vi "move calc rotation.vi"(8 "error in (no error)":errorcluster, 9 "New Value":dbl, 10 "Old Value":dbl) -> (0 "error out":errorcluster, 2 "Direction":bool=TRUE, 3 "steps":i32, 4 "Degrees":i32, 5 "rotate direction":string)   [LabVIEW 2014, in "AISAS motor.lvclass"]
uses:
  AISAS motor.lvclass
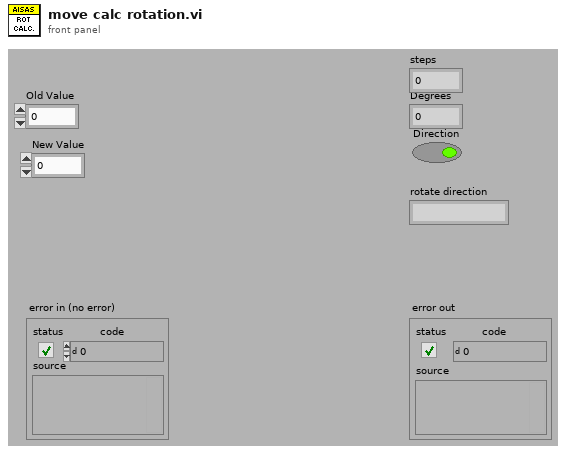
[diagram p1: front panel]
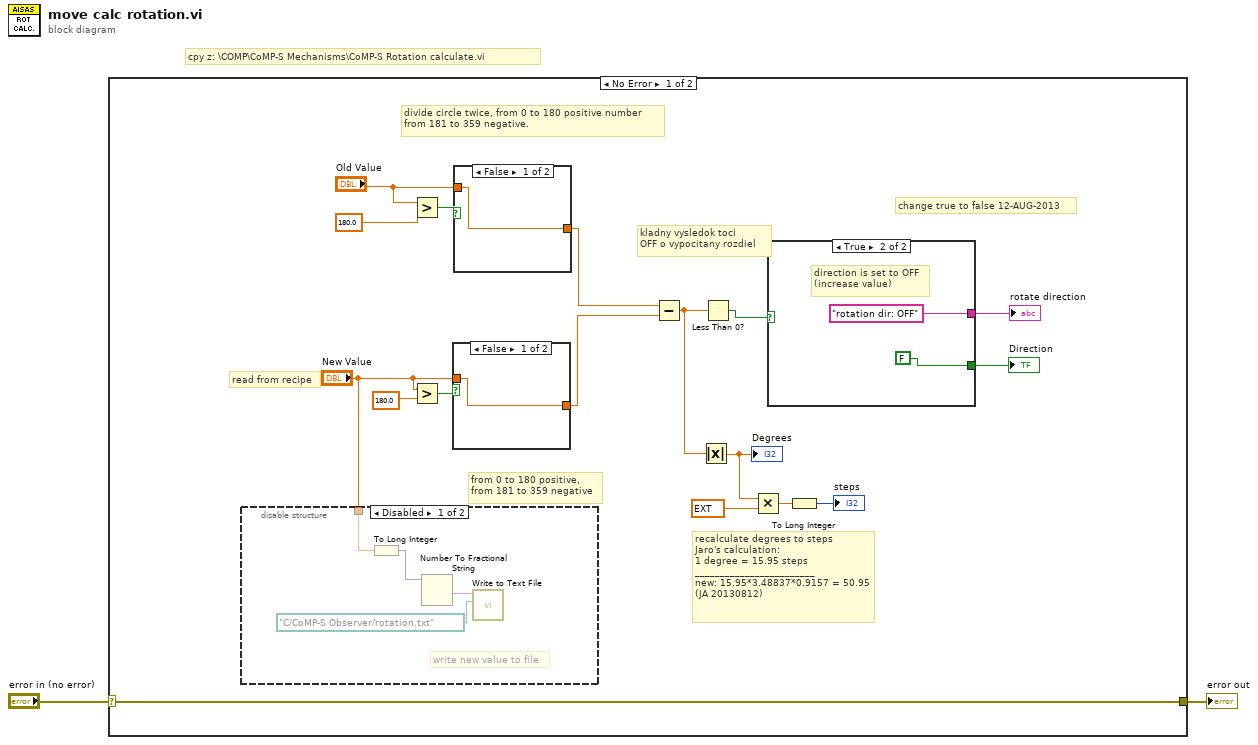
[diagram p0: block diagram]
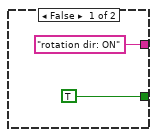
[diagram p3: hidden frame]
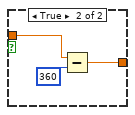
[diagram p4: hidden frame]
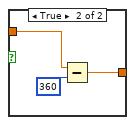
[diagram p5: hidden frame]
diagram:
  # "cpy z: \\COMP\\CoMP-S Mechanisms\\CoMP-S Rotation calculate.vi"
  n1 = case shown="No Error" "error in (no error)" {
    selector: "error in (no error)" -> [w3 w36]
    tunnel: [w3 w36] -> w1
    frame No Error {
      # "change true to false 12-AUG-2013"
      # "recalculate degrees to steps\nJaro's calculation:\n1 degree = 15.95 steps\n________________________\nnew: 15.95*3.48837*0.9157 = 50.95\n(JA 20130812)"
      # "from 0 to 180 positive, \nfrom 181 to 359 negative"
      # "divide circle twice, from 0 to 180 positive number\nfrom 181 to 359 negative."
      # "kladny vysledok toci\nOFF o vypocitany rozdiel"
      # "read from recipe"
      n2 = disable-structure shown="Disabled" {
        disable-tunnel: "New Value" -> [w23 _]
        frame Disabled {
          # "write new value to file"
          n3 = To Long Integer(number=w23) -> (32bit integer=w21:i32)
          n4 = Number To Fractional String(number=w21) -> (F-format string=w22:string)  [unwired: 3 in]
          n5 = call "Write to Text File.vi"("file path (use dialog)"=path "C:/CoMP-S Observer/rotation.txt", "text"=w22) -> ()  [unwired: 9 in, 1 out]
        }
        frame Enabled {
        }
      }
      n6 = Greater?(x="Old Value", y=180.0) -> (0:w16:bool)
      n7 = Greater?(x="New Value", y=180.0) -> (0:w15:bool)
      n8 = case shown="False" w15 {
        tunnel: "New Value" -> [w28 w30]
        tunnel: [w28 w29] -> w4
        frame False {
        }
        frame True {
          n9 = Subtract(x=w30, y=360) -> (x-y=w29:dbl)
        }
      }
      n10 = case shown="False" w16 {
        tunnel: [w32 w34] -> w14
        tunnel: "Old Value" -> [w32 w33]
        frame False {
        }
        frame True {
          n11 = Subtract(x=w33, y=360) -> (x-y=w34:dbl)
        }
      }
      n12 = Subtract(x=w14, y=w4) -> (x-y=w10:dbl)
      n13 = Absolute Value(x=w10) -> (abs(x)=w9:dbl)
      "Degrees" <- w9
      n14 = Less Than 0?(x=w10) -> (x < 0?=w13:bool)
      n15 = Multiply(x=w9, y=ext 50.95) -> (x*y=w7:ext)
      n16 = case shown="True" w13 {
        tunnel: ["rotation dir: ON" "rotation dir: OFF"] -> w12
        tunnel: [TRUE FALSE] -> w11
        frame False {
        }
        frame True {
          # "direction is set to OFF\n(increase value)"
        }
      }
      "rotate direction" <- w12
      "Direction" <- w11
      n17 = To Long Integer(number=w7) -> (32bit integer=→"steps":i32)
    }
    frame Error {
    }
  }
  "error out" <- w1
